vi "Fetch Limit Test Result.vi"(8 "error in (no error)":errorcluster, 10 "Timeout (10000 ms)":u32=10000, 11 "VISA resource name":refnum<visa-resource-name>) -> (0 "error out":errorcluster, 1 "Upper Limit Test Fail ?":bool, 2 "Lower Limit Test Fail ?":bool, 3 "VISA resource name out":refnum<visa-resource-name>)   [LabVIEW 2021, in "Agilent 532XX Series.lvlib"]
doc: "Queries and retrieves limit test results.\n\n<B>Note:</B> This VI does not check the instrument status. Typically, you call this VI only in a sequence of calls to other low-level instrument driver VIs. The sequence performs one operation. You use the low-level VIs to optimize one or more aspects of interaction with the instrument."
uses:
  <instrlib>/Agilent 532XX Series/Agilent 532XX Series.lvlib
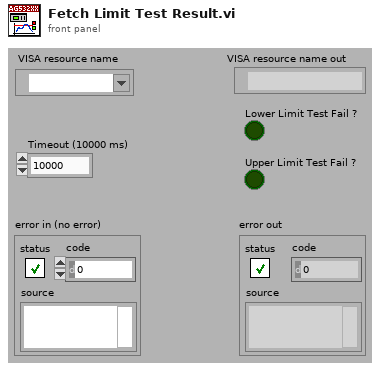
[diagram p1: front panel]
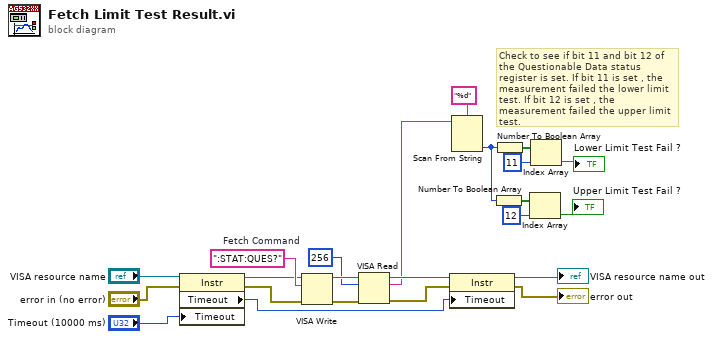
[diagram p0: block diagram]
diagram:
  w23 = ":STAT:QUES?"  # Fetch Command
  # "Check to see if bit 11 and bit 12 of the Questionable Data status register is set. If bit 11 is set , the measurement failed the lower limit test. If bit 12 is set , the measurement failed the upper limit test."
  n1 = property class="Instr"(reference="VISA resource name", error in="error in (no error)", "Timeout"="Timeout (10000 ms)") -> (reference out=w10:refnum<visa-resource-name>, error out=w11:errorcluster, "Timeout"=w12:u32)
  n2 = VISA Write(VISA resource name=w10, write buffer=w23, error in (no error)=w11) -> (VISA resource name out=w22:refnum<visa-resource-name>, error out=w21:errorcluster)  [unwired: 1 out]
  n3 = VISA Read(VISA resource name=w22, byte count=u32 256, error in (no error)=w21) -> (VISA resource name out=w16:refnum<visa-resource-name>, read buffer=w6:string, error out=w15:errorcluster)  [unwired: 1 out]
  n4 = property class="Instr"(reference=w16, error in=w15, "Timeout"=w12) -> (reference out=→"VISA resource name out":refnum<visa-resource-name>, error out=→"error out":errorcluster)
  n5 = Scan From String(format string="%d", input string=w6) -> (output 1=w3:i32)  [unwired: 2 in, 4 out]
  n6 = Number To Boolean Array(number=w3) -> (Boolean array=w5:bool[])
  n7 = Number To Boolean Array(number=w3) -> (Boolean array=w8:bool[])
  n8 = Index Array(array=w5, index=12) -> (element=→"Upper Limit Test Fail ?":bool)
  n9 = Index Array(array=w8, index=11) -> (element=→"Lower Limit Test Fail ?":bool)
